vi "TimeToSpeed (SubVI).vi"(11 "Numeric in":dbl) -> (3 "Numeric out":dbl)   [LabVIEW 2017]
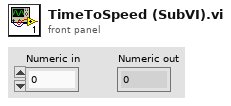
[diagram p1: front panel]
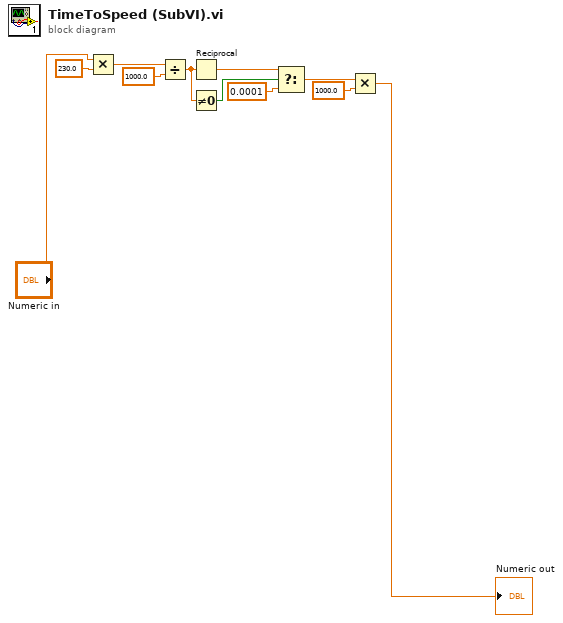
[diagram p0: block diagram]
diagram:
  n1 = Multiply(x="Numeric in", y=230.0) -> (x*y=w7:dbl)
  n2 = Divide(x=w7, y=1000.0) -> (x/y=w5:dbl)
  n3 = Reciprocal(x=w5) -> (1/x=w11:dbl)
  n4 = Not Equal To 0?(x=w5) -> (x != 0?=w10:bool)
  n5 = Select(t=w11, s=w10, f=0.0001) -> (s? t:f=w4:dbl)
  n6 = Multiply(x=w4, y=1000.0) -> (x*y=→"Numeric out":dbl)
